vi "write Error Path.vi"(8 "error in (no error)":errorcluster, 10 "Path":path, 11 "Electrometer in":refnum<class "Electrometer.lvclass">) -> (0 "error out":errorcluster, 3 "Electrometer out":refnum<class "Electrometer.lvclass">)   [LabVIEW 2016, in "Electrometer.lvclass"]
uses:
  Electrometer.lvclass
  Electrometer.lvclass/Electrometer.ctl
  ElectrometerError/ElectrometerError.lvclass
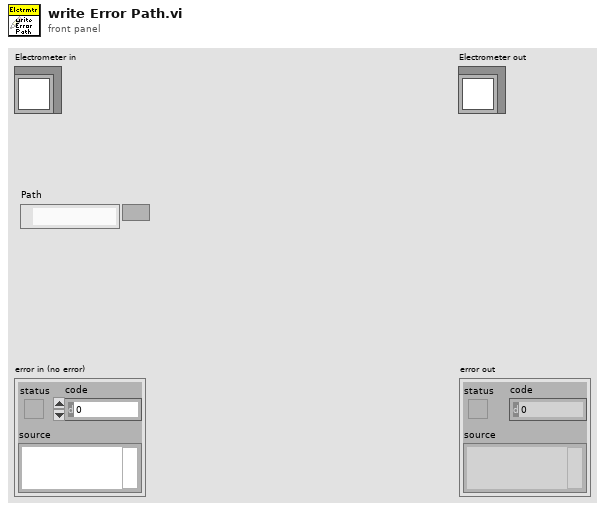
[diagram p1: front panel]
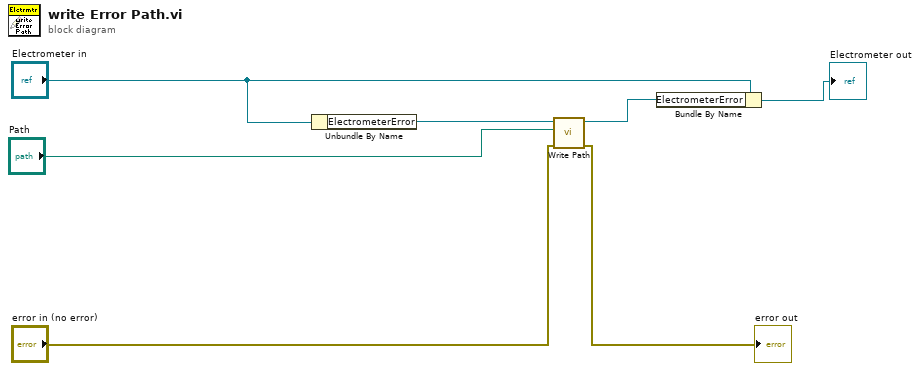
[diagram p0: block diagram]
diagram:
  n1 = Unbundle By Name("Electrometer in") -> ("ElectrometerError"=w7:refnum<class "ElectrometerError.lvclass">)
  n2 = call-dynamic "Write Path.vi"("error in (no error)"="error in (no error)", "Path"="Path", "ElectrometerError in"=w7) -> ("error out"=→"error out":errorcluster, "ElectrometerError out"=w2:refnum<class "ElectrometerError.lvclass">)  [unwired: 7 in]
  n3 = Bundle By Name(cluster="Electrometer in", "ElectrometerError"=w2) -> (→"Electrometer out":refnum<class "Electrometer.lvclass">)
